vi "to string 1.0.vi"(8 "error in (no error)":errorcluster, 10 "data in":string, 11 "Benchmark PID configuration in":refnum<class "Benchmark PID configuration.lvclass">) -> (0 "error out":errorcluster, 2 "data out":string, 3 "Benchmark PID configuration out":refnum<class "Benchmark PID configuration.lvclass">)   [LabVIEW 2018, in "Benchmark PID configuration.lvclass"]
uses:
  Benchmark PID configuration.lvclass
  Benchmark PID configuration.lvclass/Benchmark PID configuration.ctl
  <vilib>/NI/Tag Bus Module Framework/channel/TBM channel.lvclass
  <vilib>/NI/Configuration Framework/serializable configuration/NISE_CEF_serializable configuration.lvclass
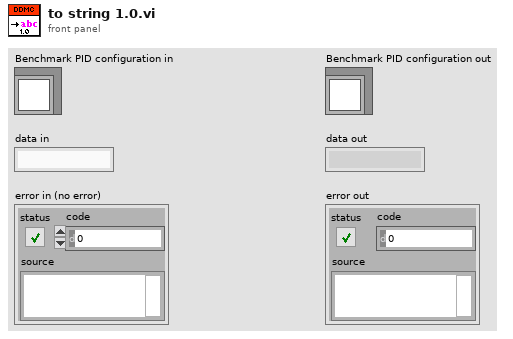
[diagram p1: front panel]
types:
  T1 = typedef "Benchmark PID configuration.lvclass/Line.ctl" = cluster{"PID Name":string, "Setpoint":refnum<class "TBM channel.lvclass">, "Variable":refnum<class "TBM channel.lvclass">, "Output":refnum<class "TBM channel.lvclass">}
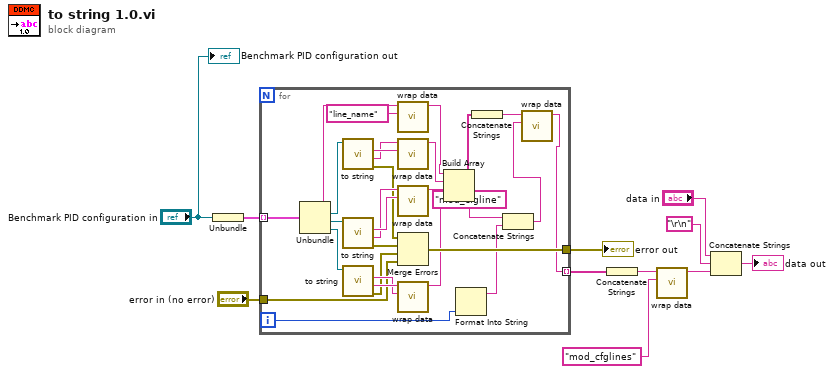
[diagram p0: block diagram]
diagram:
  n1 = Unbundle("Benchmark PID configuration in") -> (w2:T1[])
  n2 = for {
    tunnel: w2 -> [w39] mode=indexing
    tunnel: [w16] -> w3 mode=indexing
    tunnel: "error in (no error)" -> [w26]
    tunnel: [w25] -> w11
    i -> [w13]
    n3 = Unbundle(w39) -> ("PID Name"=w24:string, "Setpoint"=w34:refnum<class "TBM channel.lvclass">, "Variable"=w35:refnum<class "TBM channel.lvclass">, "Output"=w36:refnum<class "TBM channel.lvclass">)
    n4 = call-dynamic "to string.vi"("channel in"=w34) -> ("error out"=w29:errorcluster, "channel data"=w37:string, "identifier"=w38:string)  [unwired: 7 in, 1 out]
    n5 = call-dynamic "to string.vi"("channel in"=w35) -> ("error out"=w28:errorcluster, "channel data"=w30:string, "identifier"=w31:string)  [unwired: 7 in, 1 out]
    n6 = call-dynamic "to string.vi"("channel in"=w36) -> ("error out"=w27:errorcluster, "channel data"=w33:string, "identifier"=w32:string)  [unwired: 7 in, 1 out]
    n7 = call <vilib>:"wrap data.vi"("identifier"="line_name", "data to wrap"=w24) -> ("wrapped data"=w20:string)  [unwired: 9 in]
    n8 = call <vilib>:"wrap data.vi"("identifier"=w38, "data to wrap"=w37) -> ("wrapped data"=w21:string)  [unwired: 9 in]
    n9 = call <vilib>:"wrap data.vi"("identifier"=w31, "data to wrap"=w30) -> ("wrapped data"=w22:string)  [unwired: 9 in]
    n10 = Merge Errors(w29, w28, w27, w26) -> (w25:errorcluster)
    n11 = call <vilib>:"wrap data.vi"("identifier"=w32, "data to wrap"=w33) -> ("wrapped data"=w19:string)  [unwired: 9 in]
    n12 = Build Array(w20, w21, w22, w19) -> (w17:string[])
    n13 = Format Into String(w13) -> (resulting string=w14:string)  [unwired: 3 in, 1 out]
    n14 = Concatenate Strings(w17) -> (w18:string)
    n15 = Concatenate Strings("mod_cfgline" ("identifier"), w14) -> (w12:string)
    n16 = call <vilib>:"wrap data.vi"("identifier"=w12, "data to wrap"=w18) -> ("wrapped data"=w16:string)  [unwired: 9 in]
  }
  "error out" <- w11
  n17 = Concatenate Strings(w3) -> (w4:string)
  n18 = call <vilib>:"wrap data.vi"("identifier"="mod_cfglines", "data to wrap"=w4) -> ("wrapped data"=w8:string)  [unwired: 9 in]
  n19 = Concatenate Strings("data in", "\r\n", w8) -> (→"data out":string)
  "Benchmark PID configuration out" <- "Benchmark PID configuration in"
